vi "Three-PWM_Tset.vi"() -> ()   [LabVIEW 2019]
panel:
  in  "Dutycycle(%)":dbl[](array[numeric])
  in  "Error In":errorcluster
  out "Error Out":errorcluster
  in  "Stop":bool
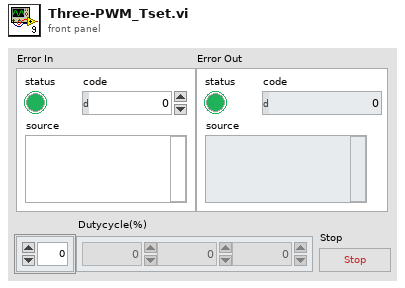
[diagram p1: front panel]
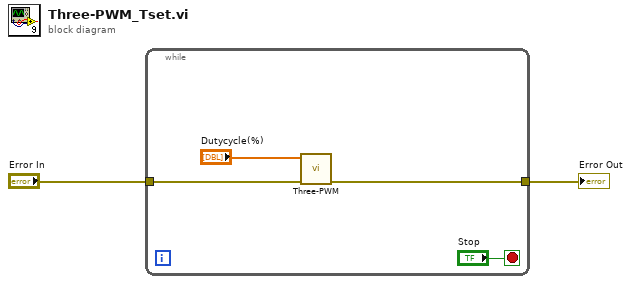
[diagram p0: block diagram]
diagram:
  n1 = while {
    tunnel: [w5] -> w2
    tunnel: "Error In" -> [w4]
    stop <- "Stop" stop-if-true
    n2 = call "Three-PWM.vi"("Error In"=w4, "Dutycycle(%)"="Dutycycle(%)") -> ("Error Out"=w5:errorcluster)  [unwired: 9 in]
  }
  "Error Out" <- w2
